vi "setPixelToColor.vi"(10 "color":u32, 11 "Pixel":u8) -> (3 "Array":u8[](array[numeric]))   [LabVIEW 2014]
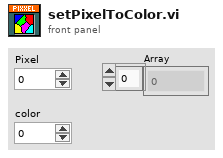
[diagram p1: front panel]
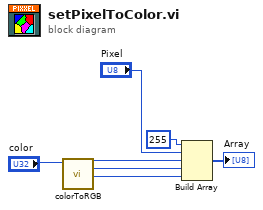
[diagram p0: block diagram]
diagram:
  n1 = call "colorToRGB.vi"("color"="color") -> ("upper limit"=w5:u8, "upper limit 3"=w7:u8, "upper limit 2"=w6:u8)  [unwired: 8 in]
  n2 = Build Array(u8 255 ("element"), "Pixel", w6, w7, w5) -> (→"Array":u8[])
